vi "PID_Discipline_WithoutSystem_1.vi"(0 "SR620_No.1_Port":refnum<visa-resource-name>="GPIB0::14::INSTR", 1 "Channel (1: A)":i32(ring)=1 items=["Ext Input", "A", "B"], 2 "SR620_No.1 (1: REF)":i32(ring) items=["A", "B", "REF", "A / B"], 3 "Meas. Mode (0: Time)":i32(ring) items=["Time", "Width", "Rise / Fall Time", "Frequency", "Period", "Phase", "Count"], 4 "Arming Mode (0: +/-time)":i32(ring)=1 items=["+/-time", "+time", "1 period", "0.01s gate", "0.1s gate", "1.0s gate", "ext trig +/- time", "ext trig +time", "ext gate/+ time/hldf", "ext triggered 1 period", "ext triggered .01s gate", "ext triggered 0.1s gate", "ext triggered 1.0s gate"], 5 "Gate Time (Auto)":dbl(ring) items=["Auto"=0.0, "1E-6"=1e-06, "2E-6"=2e-06, "5E-6"=5e-06, "1E-5"=1e-05, "2E-5"=2e-05, "5E-5"=5e-05, "1E-4"=0.0001, "2E-4"=0.0002, "5E-4"=0.0005, "1E-3"=0.001, "2E-3"=0.002, "5E-3"=0.005, ".01"=0.01, ".02"=0.02, ".05"=0.05, ".1"=0.1, ".2"=0.2, ".5"=0.5, "1"=1.0, "2"=2.0, "5"=5.0, "10"=10.0, "20"=20.0, "50"=50.0, "100"=100.0, "200"=200.0, "500"=500.0], 6 "Sample Size (1)":u32(ring)=1 items=["1"=1, "2"=2, "5"=5, "10"=10, "20"=20, "50"=50, "100"=100, "200"=200, "500"=500, "1000"=1000, "2000"=2000, "5000"=5000, "10000"=10000, "20000"=20000, "50000"=50000, "100000"=100000, "200000"=200000, "500000"=500000, "1000000"=1000000], 7 "SR620_No.1_error in (no error)1":errorcluster, 8 "Input Termination_ (0: 50 Ohms)":i32(ring) items=["50 Ohms", "1 Mohm", "UHF Prescalers"], 9 "Timeout (25000 ms)":u32=1000 step=1000, 10 "Coupling (F: DC)":bool, 11 "Ref Out (1: TTL)":i32(ring)=1 items=["ECL", "TTL"], 12 "Auto Trigger Level (True)":bool, 14 "Trigger Level (0.00 V)":dbl=0.5, 16 "Trigger Slope (T: Positive)":bool=TRUE) -> (20 "SR620_No.1":refnum<visa-resource-name>="GPIB0::15::INSTR", 27 "SR620_No1 error out":errorcluster)   [LabVIEW 2014]
doc: "Provides an example of how to use the SR620 subVIs programmatically."
uses:
  <vilib>/addons/control/pid/pid.llb/PID (DBL).vi
  <vilib>/Utility/file.llb/Write To Spreadsheet File (DBL).vi
  <vilib>/Instr/_visa.llb/VISA Configure Serial Port (Instr).vi
  <vilib>/addons/control/pid/NI_PID_pid.lvlib
panel:
  out "钟差改变量":dbl format="%#_10g"
  in  "驯服阈值(ns)":dbl=100.0
  out "驯服":bool
  out "当前粗调调整量（100ns）":i64
  in  "FPGA串口地址":refnum<visa-resource-name>="COM6"
  out "串口读取数值":i64
  out "读取缓冲区 （16进制）":string
  out "写入字符串2":string
  out "写入字符串1":string="0"
  out "最终粗调调整量（100ns）":i64
  in  "delimiter (\\n)":string="\n" caption="数据分隔符(\\n)"
  in  "文件路径: SR620_Delta_T":path=path "E:/PID_Discipline_WithoutSystem/Data/Delta_T.txt"
  out "SR620_Delta_T":dbl[](graph)
  in  "output range":cluster{"output high":dbl, "output low":dbl}={"output high"=400.0, "output low"=-400.0} caption="输出范围" {"output low" format="%.2f"; "output high" format="%.2f"}
  in  "PID gains":T1={"proportional gain (Kc)"=0.5, "integral time (Ti, min)"=0.0, "derivative time (Td, min)"=0.0} caption="PID增益" {"derivative time (Td, min)" format="%.3f"; "integral time (Ti, min)" format="%.3f"; "proportional gain (Kc)" format="%.3f"}
  out "反馈值":dbl format="%#.6f"
  in  "setpoint":dbl caption="设定值" format="%.3f"
  out "dt out (s)":dbl=1.0000000474974513 caption="dt输出(s)" format="%.3f"
  out "output":dbl caption="PID输出" format="%#.6f"
  in  "baud rate (9600) 2":u32=57600 caption="波特率(9600)"
  in  "VISA resource name 2":refnum<visa-resource-name>="COM3" caption="VISA资源名称"
  out "错误输出 2":errorcluster caption="错误输出"
  in  "baud rate (9600) 1":u32=57600 caption="波特率(9600)"
  in  "VISA resource name 1":refnum<visa-resource-name>="COM3" caption="VISA资源名称"
  out "错误输出 1":errorcluster caption="错误输出"
  out "串口工作":bool
  out "命令":string
  out "SR620_Delta_T":dbl format="%.12f"
  in  "等待时间（ms)":u32=1000
  out "总计数值":i32
  in  "?":bool
  # "串口"
  # "数据处理"
  # "钟差调整量（ns）"
  # "数据显示及波形显示区域"
  # "公共调节区域"
  # "分别设置区域"
  # "Delta_T"
  # "SR620_Delta_T"
  # "数据导出路径"
  # "SR620_Delta_T_True"
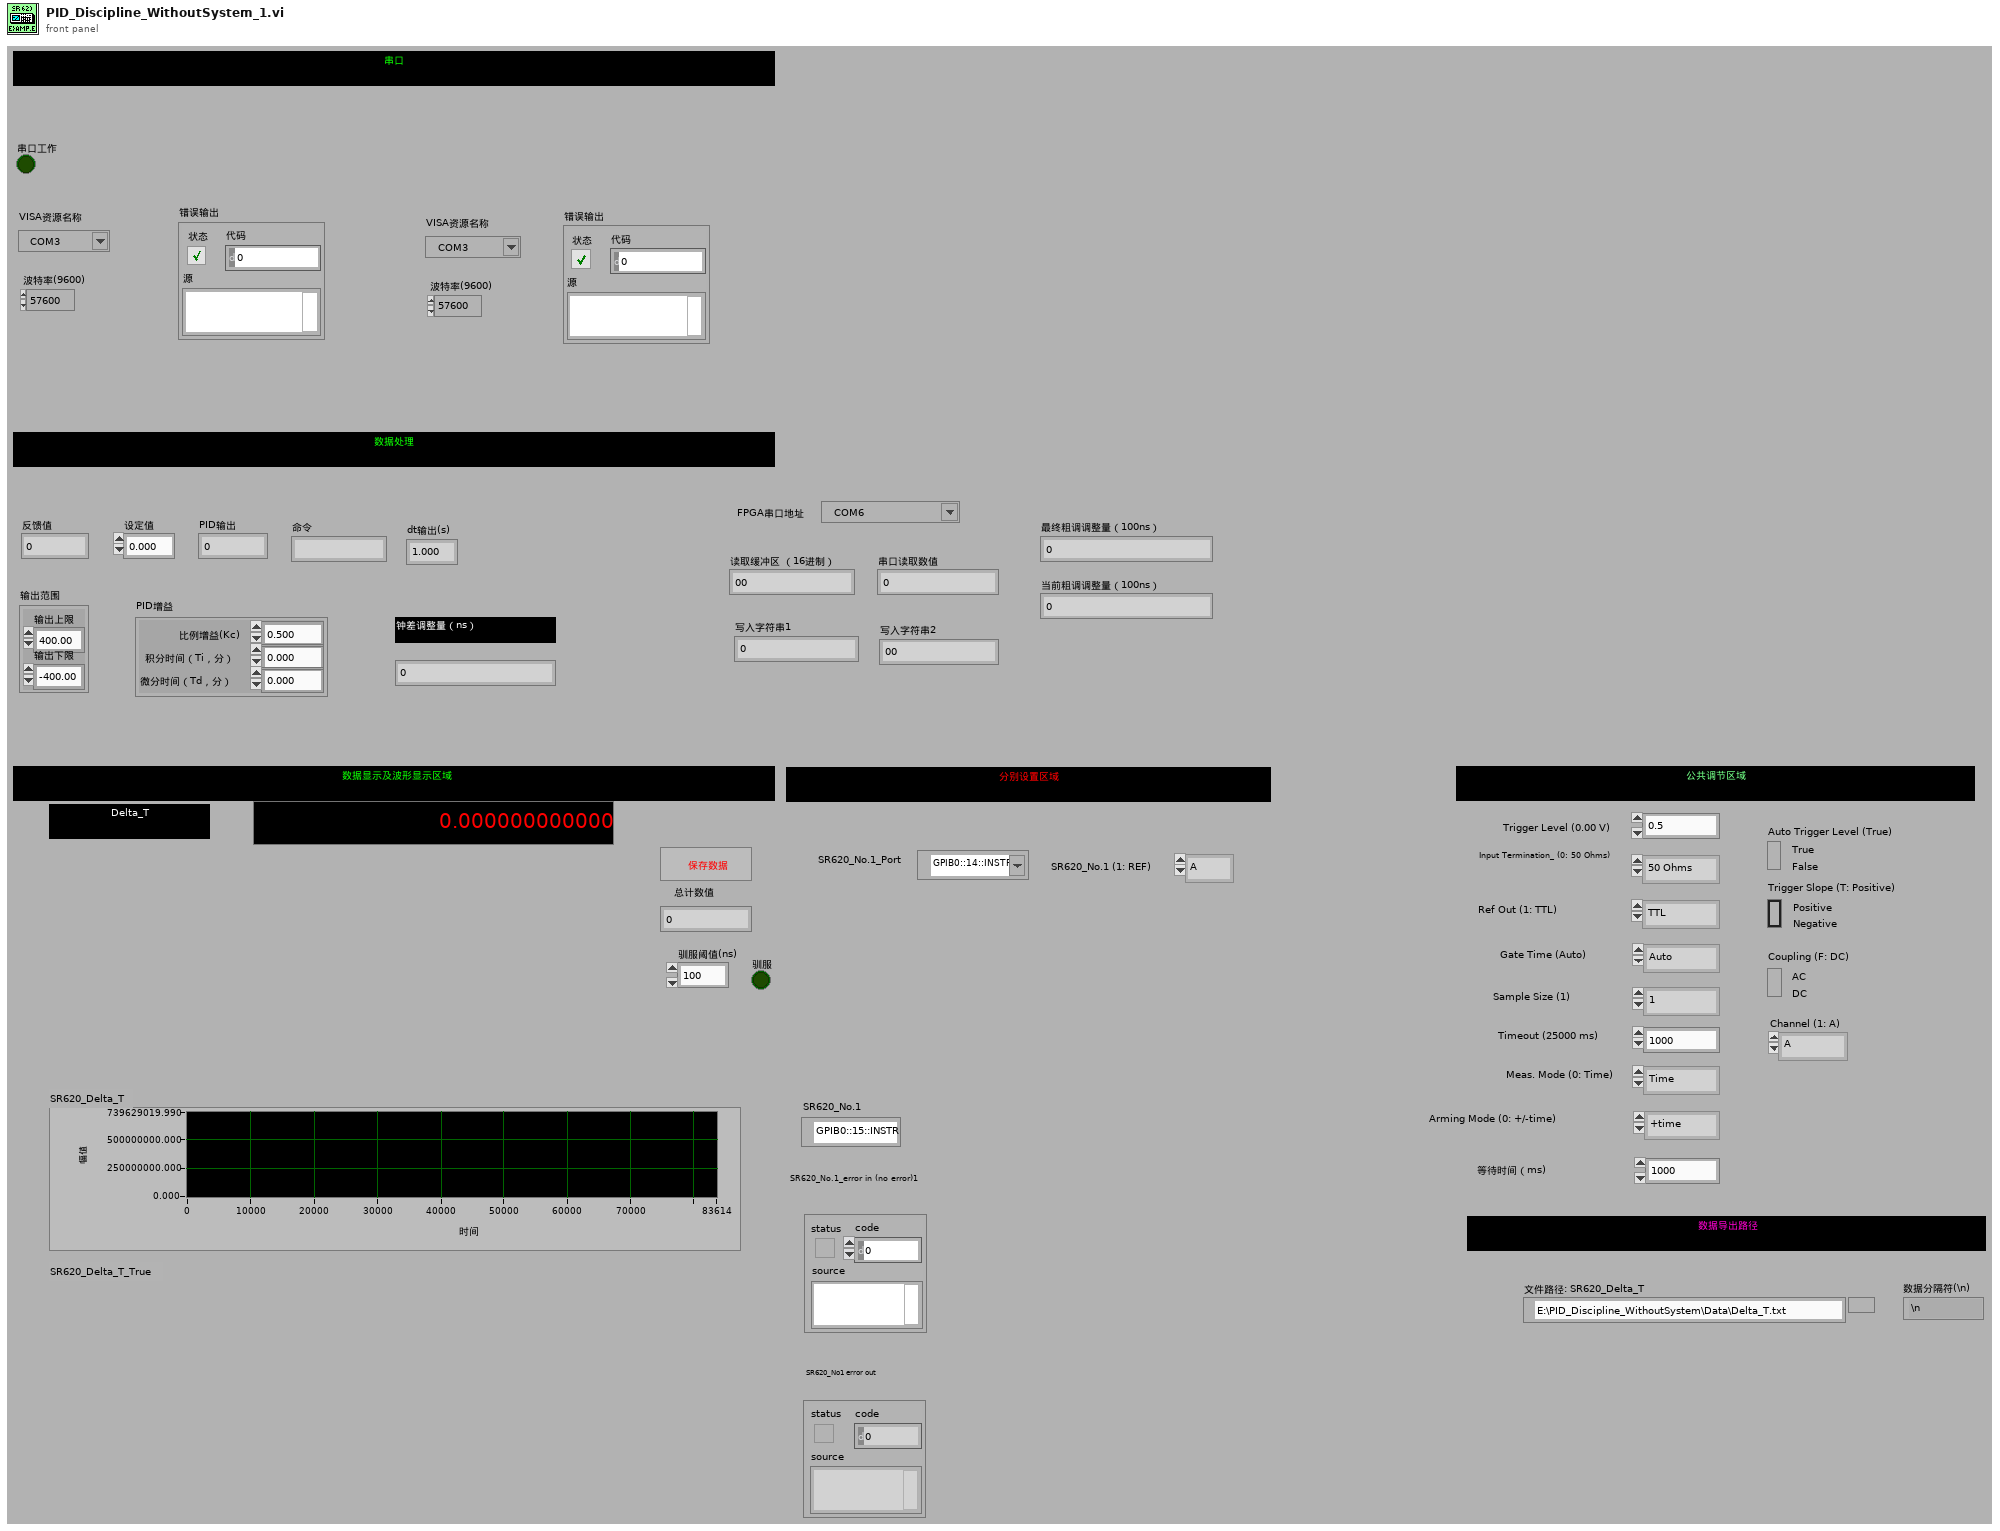
[diagram p1: front panel]
types:
  T1 = cluster{"proportional gain (Kc)":dbl, "integral time (Ti, min)":dbl, "derivative time (Td, min)":dbl}
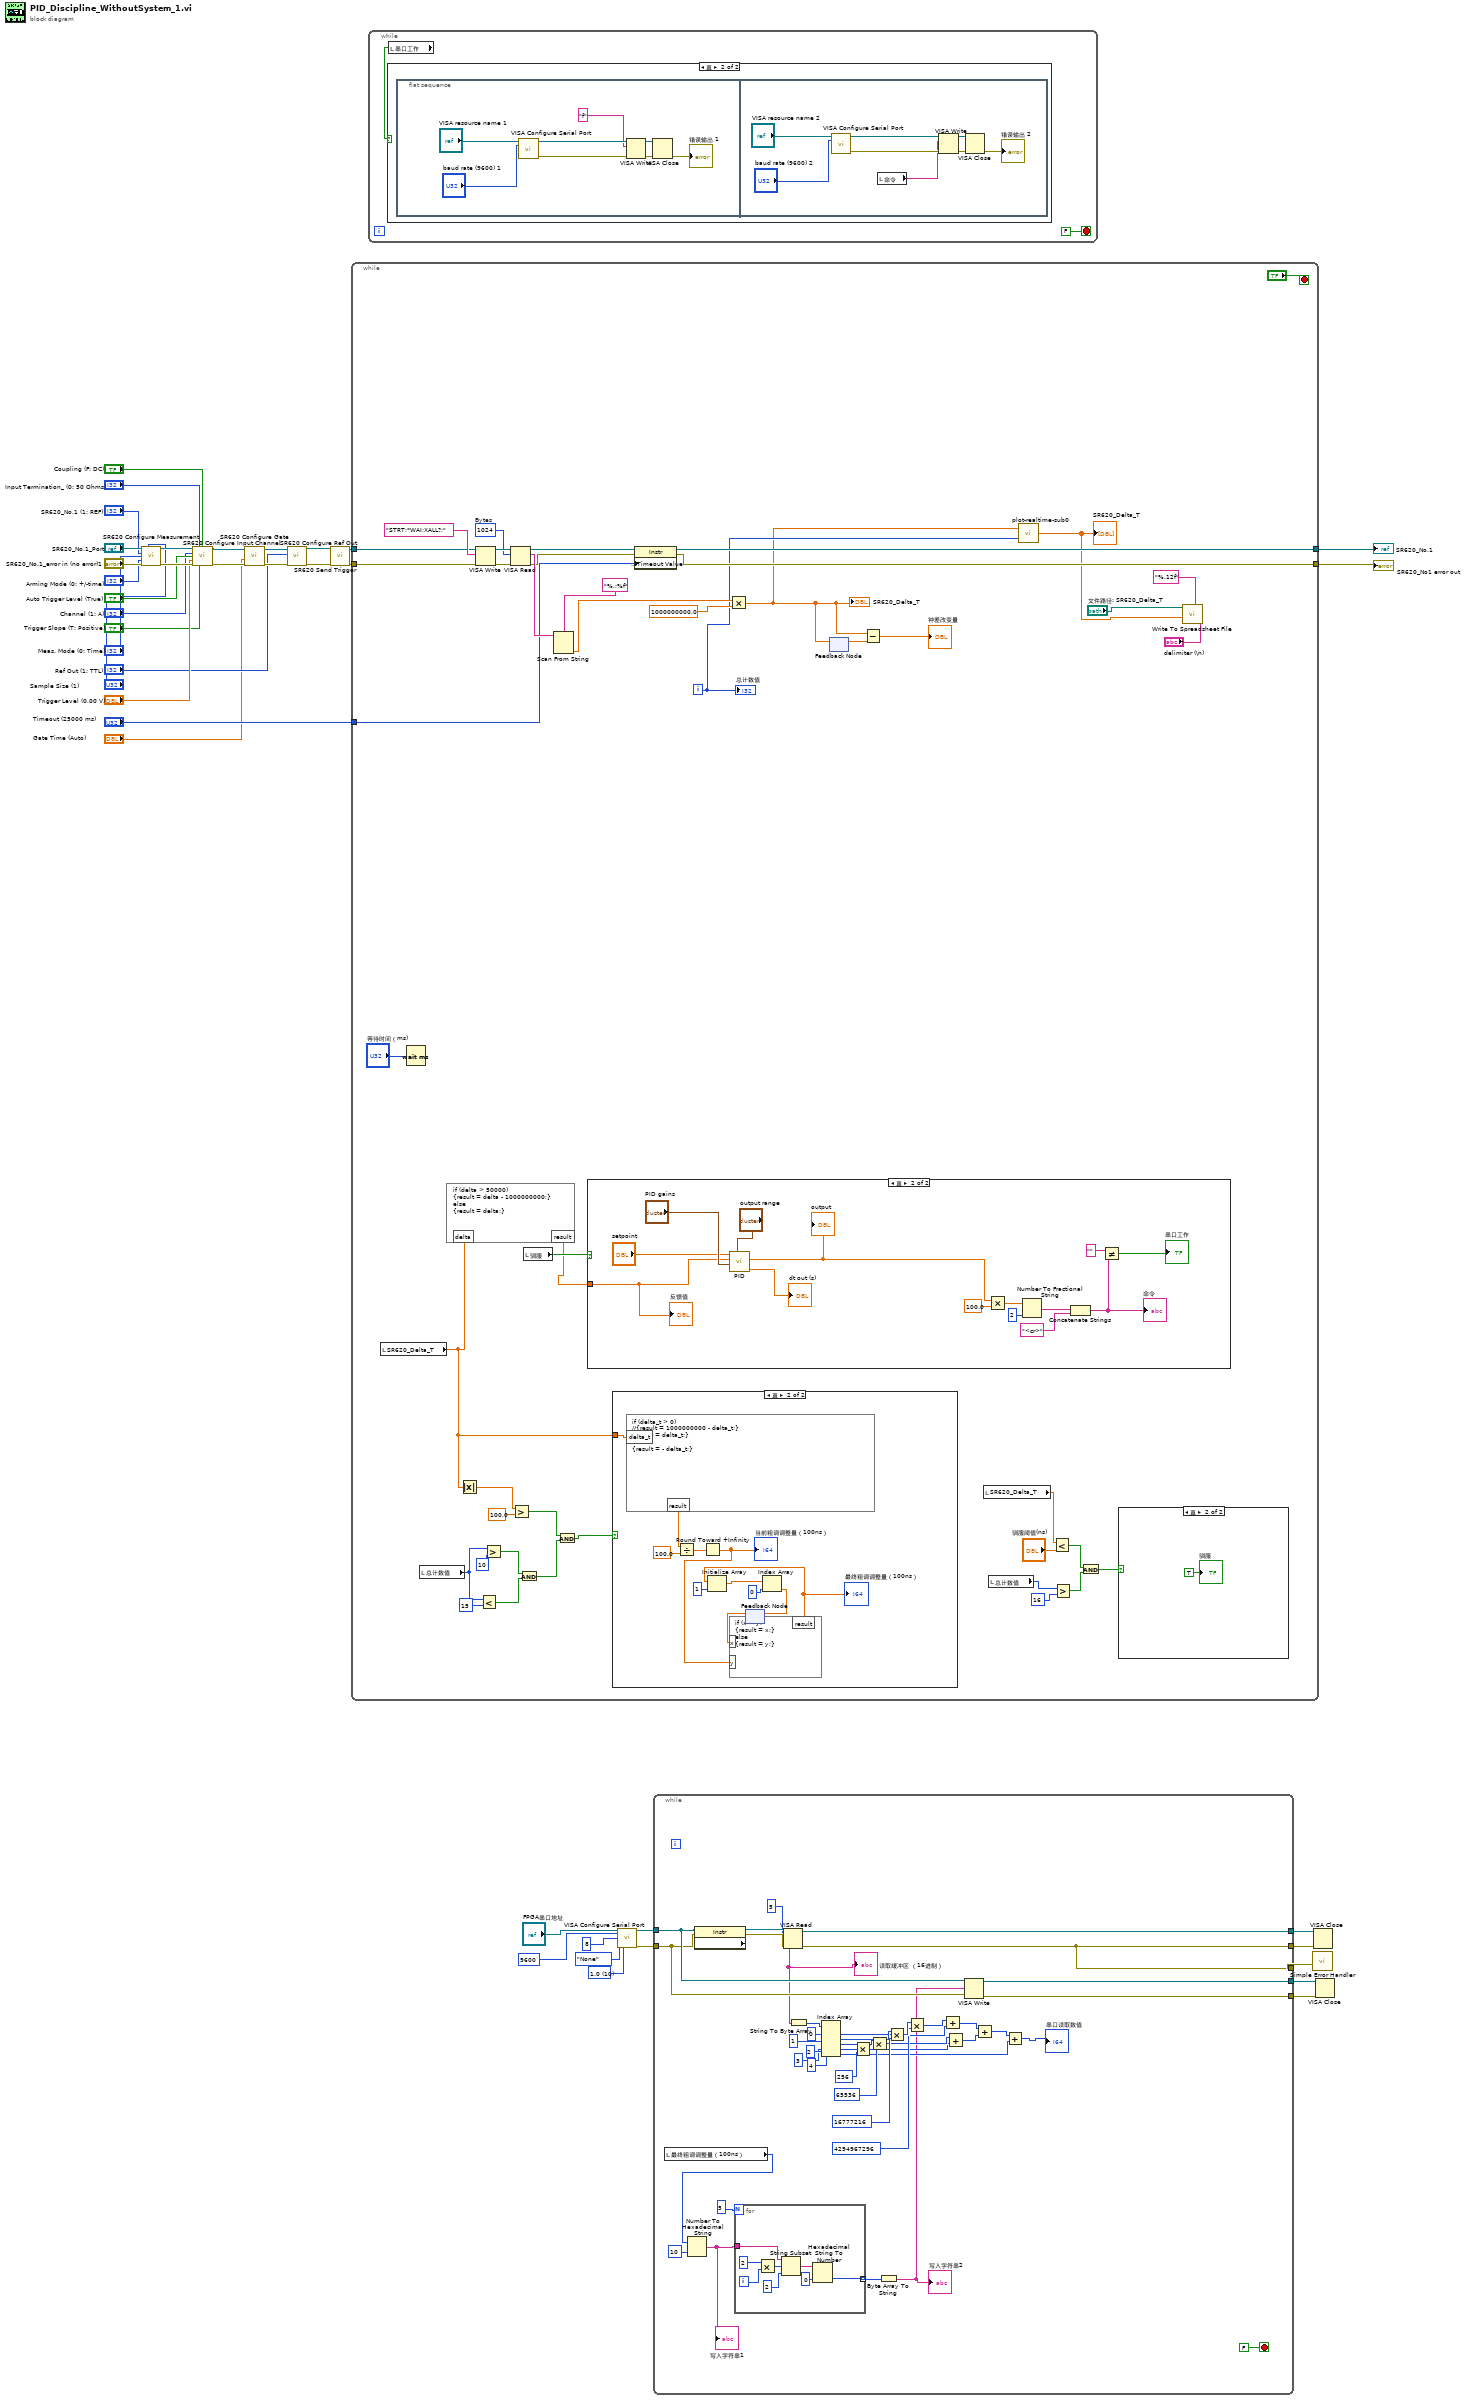
[diagram p0: block diagram]
diagram:
  w20 = u16 10 items=["1.0"=10, "1.5"=15, "2.0"=20] ("stop bits (10: 1 bit)")
  n1 = call "SR620 Configure Measurement.vi"("VISA session"="SR620_No.1_Port", "Sample Size (1)"="Sample Size (1)", "Source (2: REF)"="SR620_No.1 (1: REF)", "Measurement Mode (0: Time)"="Meas. Mode (0: Time)", "Arming Mode (0: +/-time)"="Arming Mode (0: +/-time)", "error in (no error)"="SR620_No.1_error in (no error)1") -> ("dup VISA session"=w30:refnum<visa-resource-name>, "error out"=w28:errorcluster)  [unwired: 8 in]
  n2 = call "SR620 Configure Input Channel.vi"("VISA session"=w30, "Input Termination (0: 50 Ohms)"="Input Termination_ (0: 50 Ohms)", "Coupling (F: DC)"="Coupling (F: DC)", "Channel (1: A)"="Channel (1: A)", "Auto Trigger Level (True)"="Auto Trigger Level (True)", "Trigger Level (0.00 V)"="Trigger Level (0.00 V)", "error in (no error)"=w28, "Trigger Slope (T: Positive)"="Trigger Slope (T: Positive)") -> ("dup VISA session"=w29:refnum<visa-resource-name>, "error out"=w27:errorcluster)  [unwired: 6 in]
  n3 = call "SR620 Configure Gate.vi"("error in (no error)"=w27, "Gate Time (Auto)"="Gate Time (Auto)", "VISA session"=w29) -> ("error out"=w32:errorcluster, "dup VISA session"=w31:refnum<visa-resource-name>)  [unwired: 5 in]
  n4 = call "SR620 Configure Ref Out.vi"("error in (no error)"=w32, "Amplitude: Ref Output (1: TTL)"="Ref Out (1: TTL)", "VISA session"=w31) -> ("error out"=w33:errorcluster, "dup VISA session"=w34:refnum<visa-resource-name>)  [unwired: 3 in]
  n5 = call "SR620 Send Trigger.vi"("VISA session"=w34, "error in (no error)"=w33) -> ("dup VISA session"=w38:refnum<visa-resource-name>, "error out"=w37:errorcluster)  [unwired: 12 in]
  n6 = while "While循环" {
    tunnel: w38 -> [w75]
    tunnel: w37 -> [w74]
    tunnel: "Timeout (25000 ms)" -> [w46]
    tunnel: [w73] -> w25
    tunnel: [w72] -> w24
    i -> [w45]
    stop <- "?" stop-if-true
    w81 = u32 1024  # Bytes
    n7 = local read "SR620_Delta_T"() -> (w40:dbl)
    n8 = Wait (ms)(milliseconds to wait="等待时间（ms)") -> ()  [unwired: 1 out]
    n9 = local read "总计数值"() -> (w62:i32)
    n10 = formula code="if (delta > 50000)\n{result = delta - 1000000000;}\nelse\n{result = delta;}"("delta"=w40) -> ("result"=w48:dbl)
    n11 = Absolute Value(x=w40) -> (abs(x)=w47:dbl)
    n12 = VISA Write(VISA resource name=w75, write buffer="STRT;*WAI;XALL?;" ("write buffer (\"\")"), error in (no error)=w74) -> (VISA resource name out=w82:refnum<visa-resource-name>, error out=w83:errorcluster)  [unwired: 1 out]
    n13 = Less?(x=w62, y=15) -> (x < y?=w59:bool)
    n14 = Greater?(x=w62, y=10) -> (0:w60:bool)
    n15 = VISA Read(VISA resource name=w82, byte count=w81, error in (no error)=w83) -> (VISA resource name out=w77:refnum<visa-resource-name>, read buffer=w78:string, error out=w76:errorcluster)  [unwired: 1 out]
    n16 = Greater?(x=w47, y=100.0) -> (0:w58:bool)
    n17 = And(x=w60, y=w59) -> (x .and. y?=w57:bool)
    n18 = local read "驯服"() -> (w50:bool)
    n19 = Scan From String(format string="%.;%f", input string=w78) -> (output 1=w70:dbl)  [unwired: 3 in, 3 out]
    n20 = And(x=w58, y=w57) -> (x .and. y?=w56:bool)
    n21 = case shown="真" w50 {
      tunnel: w48 -> [_ w106]
      frame False {
      }
      frame True {
        n22 = call-poly <vilib>:"PID.vi"("output range"="output range", "PID gains"="PID gains", "process variable"=w106, "setpoint"="setpoint") -> ("dt out (s)"=→"dt out (s)":dbl, "output"=w98:dbl)  [unwired: 6 in]
        "output" <- w98
        n23 = Multiply(x=w98, y=100.0) -> (x*y=w97:dbl)
        n24 = Number To Fractional String(number=w97, precision (6)=i16 2 ("精度(6)")) -> (F-format string=w104:string)  [unwired: 2 in]
        n25 = Concatenate Strings(w104, "<cr>" ("字符串")) -> (w100:string)
        "命令" <- w100
        n26 = Not Equal?(x="", y=w100) -> (x != y?=→"串口工作":bool)
        "反馈值" <- w106
      }
    }
    n27 = case shown="真" w56 {
      tunnel: w40 -> [_ w86]
      frame False {
      }
      frame True {
        n28 = formula code="if (delta_t > 0)\n//{result = 1000000000 - delta_t;}\n{result = delta_t;}\nelse\n{result = - delta_t;}"("delta_t"=w86) -> ("result"=w95:dbl)
        n29 = Divide(x=w95, y=100.0) -> (x/y=w94:dbl)
        n30 = Round Toward +Infinity(x=w94) -> (ceil(x): smallest int >= x=w88:dbl)
        "当前粗调调整量（100ns）" <- w88
        n31 = feedback #1() -> (w89:dbl)  [unwired: 1 in]
        n32 = formula code="if (x > y)\n{result = x;}\nelse\n{result = y;}"("x"=w89, "y"=w88) -> ("result"=w87:dbl)
        "最终粗调调整量（100ns）" <- w87
        n33 = Initialize Array(w87, 1 ("维数大小")) -> (w91:dbl[])
        n34 = Index Array(array=w91, index=0 ("索引")) -> (element=w90:dbl)
        n35 = feedback-in #1(w90) -> ()
      }
    }
    n36 = property class="Instr"(reference=w77, error in=w76, "General Settings:Timeout Value"=w46) -> (reference out=w73:refnum<visa-resource-name>, error out=w72:errorcluster)
    n37 = Multiply(x=w70, y=1000000000.0) -> (x*y=w44:dbl)
    "SR620_Delta_T" <- w44
    n38 = feedback #2() -> (w43:dbl)  [unwired: 1 in]
    n39 = feedback-in #2(w44) -> ()
    n40 = Subtract(x=w44, y=w43) -> (x-y=→"钟差改变量":dbl)
    n41 = local read "SR620_Delta_T"() -> (w41:dbl)
    n42 = local read "总计数值"() -> (w55:i32)
    n43 = call "plot-realtime-sub0.vi"("索引"=w45, "x"=w44) -> ("数组"=w67:dbl[])
    "SR620_Delta_T" <- w67
    n44 = Less?(x=w41, y="驯服阈值(ns)") -> (x < y?=w53:bool)
    n45 = Greater?(x=w55, y=16) -> (0:w52:bool)
    n46 = And(x=w53, y=w52) -> (x .and. y?=w51:bool)
    n47 = case shown="真" w51 {
      frame False {
      }
      frame True {
        "驯服" <- TRUE
      }
    }
    n48 = call-poly <vilib>:"Write To Spreadsheet File.vi"("delimiter (\\t)"="delimiter (\\n)", "format (%.3f)"="%.12f", "1D data"=w67, "file path (dialog if empty)"="文件路径: SR620_Delta_T") -> ()  [unwired: 4 in, 1 out]
    "总计数值" <- w45
  }
  "SR620_No.1" <- w25
  "SR620_No1 error out" <- w24
  n49 = while {
    stop <- FALSE stop-if-true
    n50 = local read "串口工作"() -> (w111:bool)
    n51 = case shown="真" w111 {
      frame False {
      }
      frame True {
        n52 = flat-sequence {
          frame #0 {
            n53 = call-poly "VISA Configure Serial Port"("VISA resource name"="VISA resource name 1", "baud rate (9600)"="baud rate (9600) 1") -> ("VISA resource name out"=w120:refnum<visa-resource-name>, "error out"=w116:errorcluster)  [unwired: 12 in]
            n54 = VISA Write(VISA resource name=w120, write buffer="f" ("写入缓冲区"), error in (no error)=w116) -> (VISA resource name out=w117:refnum<visa-resource-name>, error out=w115:errorcluster)  [unwired: 1 out]
            n55 = VISA Close(VISA resource name=w117, error in (no error)=w115) -> (error out=→"错误输出 1":errorcluster)
          }
          frame #1 {
            n56 = call-poly "VISA Configure Serial Port"("VISA resource name"="VISA resource name 2", "baud rate (9600)"="baud rate (9600) 2") -> ("VISA resource name out"=w122:refnum<visa-resource-name>, "error out"=w125:errorcluster)  [unwired: 12 in]
            n57 = local read "命令"() -> (w121:string)
            n58 = VISA Write(VISA resource name=w122, write buffer=w121, error in (no error)=w125) -> (VISA resource name out=w124:refnum<visa-resource-name>, error out=w126:errorcluster)  [unwired: 1 out]
            n59 = VISA Close(VISA resource name=w124, error in (no error)=w126) -> (error out=→"错误输出 2":errorcluster)
          }
        }
      }
    }
  }
  n60 = call-poly "VISA Configure Serial Port"("VISA resource name"="FPGA串口地址", "baud rate (9600)"=u32 9600, "data bits (8)"=u16 8, "parity (0:none)"=enum16{"None", "Odd", "Even", "Mark", "Space"}."None", "stop bits (10: 1 bit)"=w20) -> ("VISA resource name out"=w18:refnum<visa-resource-name>, "error out"=w17:errorcluster)  [unwired: 9 in]
  n61 = while {
    tunnel: w18 -> [w166]
    tunnel: w17 -> [w165]
    tunnel: [w163] -> w16
    tunnel: [w162] -> w15
    tunnel: [w162] -> w14
    tunnel: [w161] -> w13
    tunnel: [w160] -> w12
    stop <- FALSE stop-if-true
    n62 = local read "最终粗调调整量（100ns）"() -> (w130:i64)
    n63 = Number To Hexadecimal String(1:i16 10 ("宽度(-)"), 2:w130) -> (0:w132:string)
    "写入字符串1" <- w132
    n64 = property class="Instr" props=["Serial Settings:Number of Bytes at Serial Port"](reference=w166, error in=w165) -> (reference out=w168:refnum<visa-resource-name>, error out=w167:errorcluster)  [unwired: 1 out]
    n65 = for {
      N: 5 -> [_]
      tunnel: w132 -> [w172]
      tunnel: [w169] -> w134 mode=indexing
      i -> [w176]
      n66 = Multiply(x=2, y=w176) -> (x*y=w174:i32)
      n67 = String Subset(string=w172, offset (0)=w174, length (rest)=2) -> (substring=w171:string)
      n68 = Hexadecimal String To Number(string=w171, default (0uL)=u8 0 ("默认(0 U32)")) -> (number=w169:u8)  [unwired: 1 in, 1 out]
    }
    n69 = VISA Read(VISA resource name=w168, byte count=5, error in (no error)=w167) -> (VISA resource name out=w163:refnum<visa-resource-name>, read buffer=w136:string, error out=w162:errorcluster)  [unwired: 1 out]
    "读取缓冲区 （16进制）" <- w136
    n70 = String To Byte Array(string=w136) -> (unsigned byte array=w159:u8[])
    n71 = Index Array ("索引数组")(array=w159, index #1=0 ("索引"), index #2=1 ("索引"), index #3=2 ("索引"), index #4=3 ("索引"), index #5=4 ("索引")) -> (element #1=w147:u8, element #2=w148:u8, element #3=w150:u8, element #4=w151:u8, element #5=w138:u8)
    n72 = Multiply ("乘")(x=w151, y=i64 256) -> (x*y=w142:i64)
    n73 = Multiply ("乘")(x=w150, y=i64 65536) -> (x*y=w143:i64)
    n74 = Byte Array To String(unsigned byte array=w134) -> (string=w131:string)
    "写入字符串2" <- w131
    n75 = Multiply ("乘")(x=w148, y=i64 16777216) -> (x*y=w144:i64)
    n76 = Multiply ("乘")(x=w147, y=i64 4294967296) -> (x*y=w145:i64)
    n77 = Add ("加")(x=w145, y=w144) -> (x+y=w141:i64)
    n78 = Add ("加")(x=w143, y=w142) -> (x+y=w140:i64)
    n79 = VISA Write(VISA resource name=w166, write buffer=w131, error in (no error)=w165) -> (VISA resource name out=w161:refnum<visa-resource-name>, error out=w160:errorcluster)  [unwired: 1 out]
    n80 = Add ("加")(x=w141, y=w140) -> (x+y=w139:i64)
    n81 = Add ("加")(x=w139, y=w138) -> (x+y=→"串口读取数值":i64)
  }
  n82 = call <vilib>:"Simple Error Handler.vi"("error in (no error)"=w14) -> ()  [unwired: 4 in, 5 out]
  n83 = VISA Close(VISA resource name=w16, error in (no error)=w15) -> ()  [unwired: 1 out]
  n84 = VISA Close(VISA resource name=w13, error in (no error)=w12) -> ()  [unwired: 1 out]
